vi "tdms查看.vi"(11 "路径":path) -> ()   [LabVIEW 2012]
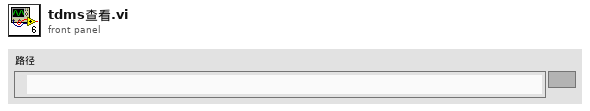
[diagram p1: front panel]
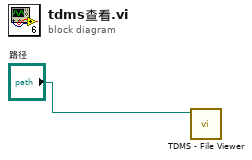
[diagram p0: block diagram]
diagram:
  n1 = call <vilib>:"TDMS - File Viewer.vi"("file path"="路径") -> ()  [unwired: 5 in, 2 out]
